vi "alapértelmezett előlap.vi"(3 "error in (no error)":errorcluster, 7 "VI Reference":refnum<vi>, 9 "Application reference":refnum<vi>, 10 "Pane Control":refnum<vi>, 11 "TabControl in":refnum<vi>) -> (0 "error out":errorcluster)   [LabVIEW 2016]
doc: "Ez a VI arra való, hogy a program futtatásakor az 1-es TAB control köré korlátozódjon a front panel."
uses:
  <vilib>/Utility/miscctls.llb/LVPointTypeDef.ctl
  <vilib>/Utility/miscctls.llb/LVRectTypeDef.ctl
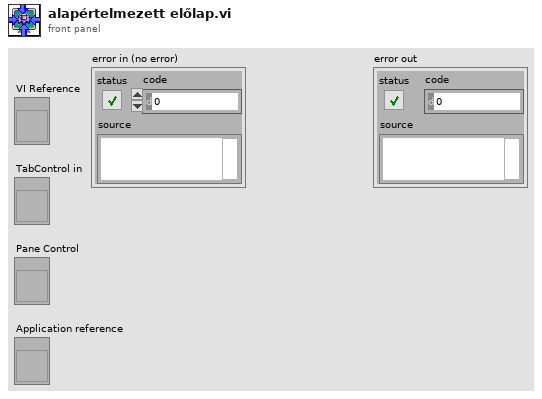
[diagram p1: front panel]
types:
  T1 = typedef "LVRectTypeDef.ctl" = cluster{"Left":i16, "Top":i16, "Right":i16, "Bottom":i16}
  T2 = typedef "LVPointTypeDef.ctl" = cluster{"Horizontal":i16, "Vertical":i16}
  T3 = typedef "LVBoundsTypeDef.ctl" = cluster{"Width":u32, "Height":u32}
  T4 = typedef "LVAllMonitorsDisplayTypeDef.ctl" = cluster{"Bounds":cluster{"Left":i16, "Top":i16, "Right":i16, "Bottom":i16}, "Depth":i16}[]
  T5 = cluster{"Bounds":cluster{"Left":i16, "Top":i16, "Right":i16, "Bottom":i16}, "Depth":i16}
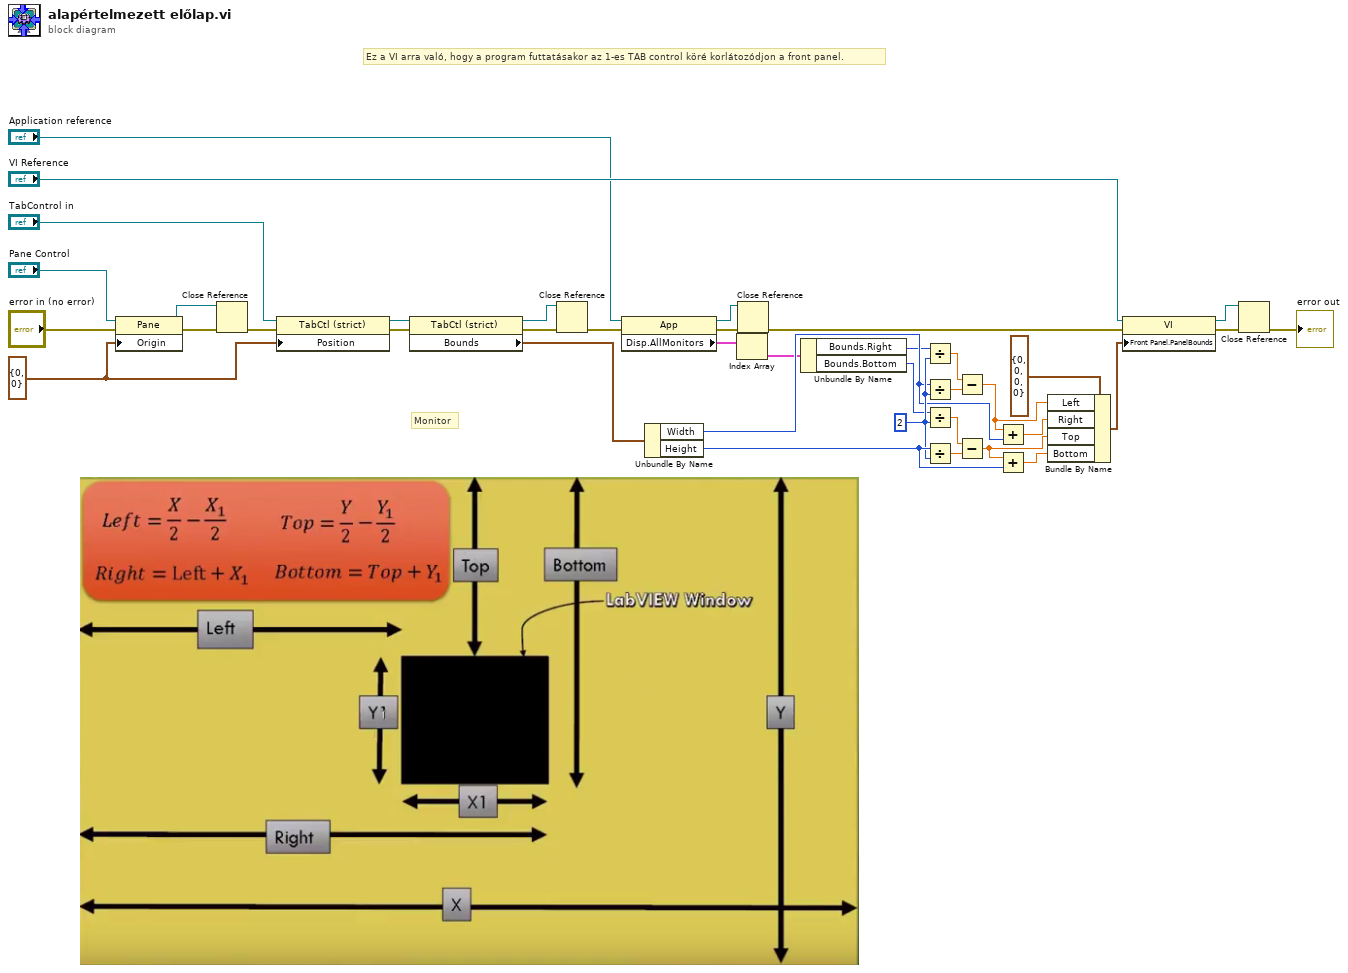
[diagram p0: block diagram]
diagram:
  w29 = i16 2 ("y")
  w15 = T2 {"Horizontal"=0, "Vertical"=0} ("Origin")
  # "Monitor"
  # "Ez a VI arra való, hogy a program futtatásakor az 1-es TAB control köré korlátozódjon a front panel."
  n1 = property on="Property Node" class="Pane"(reference="Pane Control", error in="error in (no error)", "Origin"=w15) -> (reference out=w6:refnum<vi>, error out=w5:errorcluster)
  n2 = Close Reference(reference=w6, error in (no error)=w5) -> (error out=w1:errorcluster)
  n3 = property on="Property Node" class="TabCtl (strict)"(reference="TabControl in", error in=w1, "Position"=w15) -> (reference out=w17:refnum<vi>, error out=w18:errorcluster)
  n4 = property on="Property Node" class="TabCtl (strict)"(reference=w17, error in=w18) -> (reference out=w8:refnum<vi>, error out=w7:errorcluster, "Bounds"=w19:T3)
  n5 = Close Reference(reference=w8, error in (no error)=w7) -> (error out=w2:errorcluster)
  n6 = property class="App"(reference="Application reference", error in=w2) -> (reference out=w12:refnum<vi>, error out=w11:errorcluster, "Disp.AllMonitors"=w20:T4)
  n7 = Unbundle By Name(w19) -> ("Width"=w27:u32, "Height"=w30:u32)
  n8 = Index Array(array=w20) -> (element=w21:T5)  [unwired: 1 in]
  n9 = Close Reference(reference=w12, error in (no error)=w11) -> (error out=w3:errorcluster)
  n10 = Unbundle By Name(w21) -> ("Bounds.Right"=w22:i16, "Bounds.Bottom"=w23:i16)
  n11 = Divide(x=w22, y=w29) -> (x/y=w24:dbl)
  n12 = Divide(x=w27, y=w29) -> (x/y=w25:dbl)
  n13 = Divide(x=w23, y=w29) -> (x/y=w26:dbl)
  n14 = Divide(x=w30, y=w29) -> (x/y=w28:dbl)
  n15 = Subtract(x=w24, y=w25) -> (x-y=w34:dbl)
  n16 = Subtract(x=w26, y=w28) -> (x-y=w36:dbl)
  n17 = Add(x=w34, y=w27) -> (x+y=w35:dbl)
  n18 = Add(x=w36, y=w30) -> (x+y=w37:dbl)
  n19 = Bundle By Name(cluster=T1 {"Left"=0, "Top"=0, "Right"=0, "Bottom"=0} ("Front Panel Window:Panel Bounds"), "Left"=w34, "Right"=w35, "Top"=w36, "Bottom"=w37) -> (w38:T1)
  n20 = property on="Property Node" class="VI"(reference="VI Reference", error in=w3, "Front Panel.PanelBounds"=w38) -> (reference out=w9:refnum<vi>, error out=w10:errorcluster)
  n21 = Close Reference(reference=w9, error in (no error)=w10) -> (error out=→"error out":errorcluster)
